vi "ReinitialControls.vi"(8 "error in (no error)":errorcluster, 11 "Control reference Array":refnum<vi>[](array[refnum])) -> (0 "error out":errorcluster)   [LabVIEW 2017]
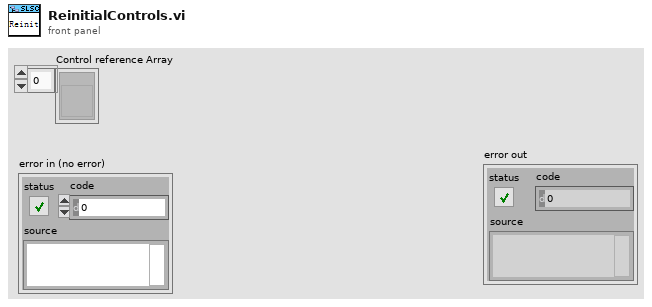
[diagram p1: front panel]
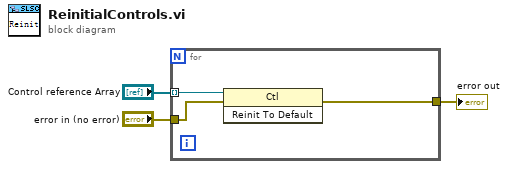
[diagram p0: block diagram]
diagram:
  n1 = for {
    tunnel: "Control reference Array" -> [w6] mode=indexing
    tunnel: "error in (no error)" -> [w5]
    tunnel: [w4] -> w1
    n2 = invoke class="Ctl" method="Reinit To Default"(reference=w6, error in=w5) -> (error out=w4:errorcluster)  [unwired: 1 in, 2 out]
  }
  "error out" <- w1
